vi "Lang Set Image Page.vi"(8 "error in (no error)":errorcluster, 10 "Image":T1, 11 "Configuration Window in":refnum<class "Configuration Window.lvclass">) -> (0 "error out":errorcluster, 3 "Configuration Window out":refnum<class "Configuration Window.lvclass">)   [LabVIEW 2018, in "Configuration Window.lvlib" / "Configuration Window.lvclass"]
uses:
  Configuration Window.lvclass
  Framework/Framework/Const Lang CfgWnd Image.ctl
  Framework/Framework/Const Lang Property.ctl
  Configuration Window.lvclass/Configuration Window.ctl
  Framework/Framework/Framework.lvclass
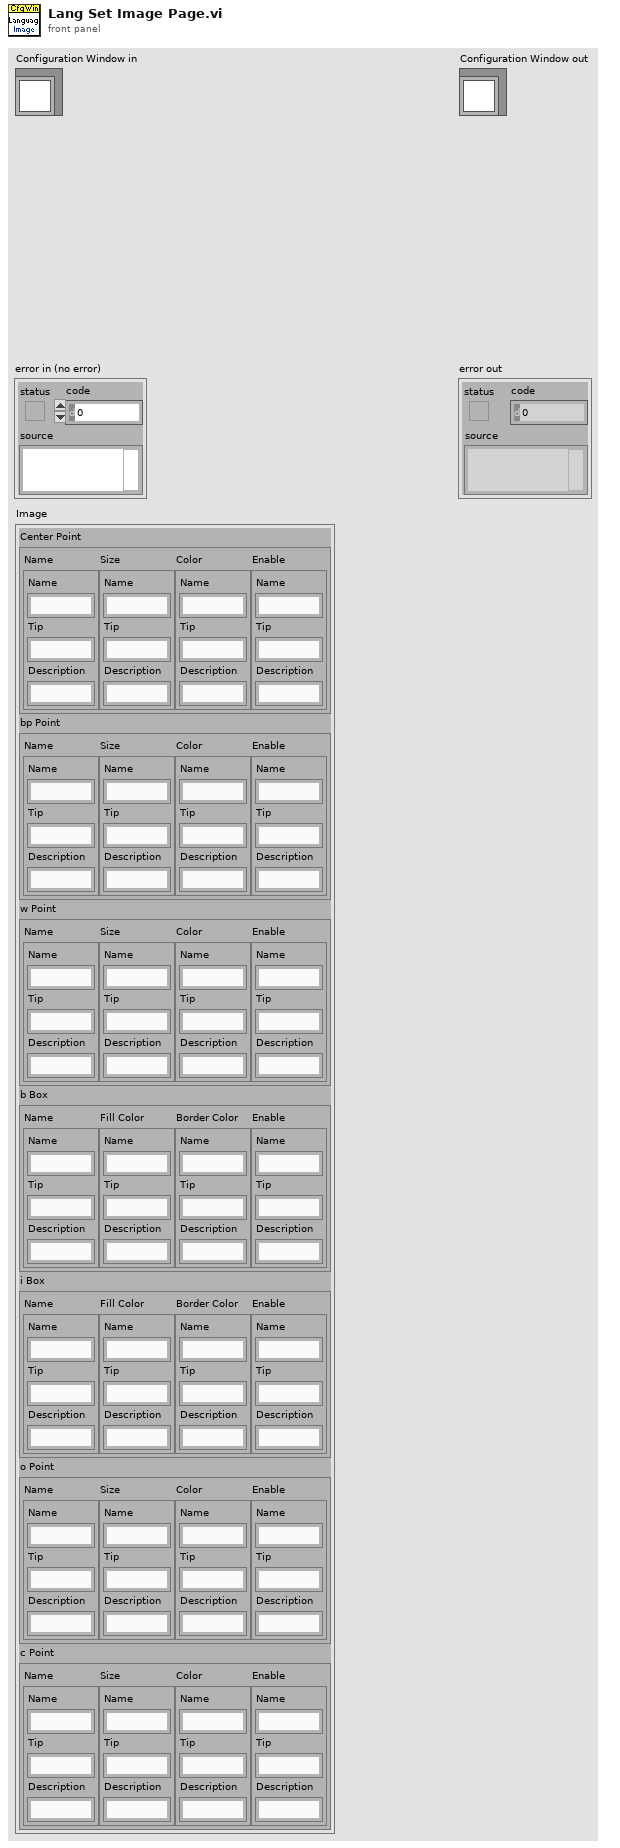
[diagram p1: front panel]
types:
  T1 = typedef "Framework.lvlib/Framework.lvclass/Const Lang CfgWnd Image.ctl" = cluster{"Center Point":cluster{"Name":T2, "Size":T2, "Color":T2, "Enable":T2}, "bp Point":cluster{"Name":T2, "Size":T2, "Color":T2, "Enable":T2}, "w Point":cluster{"Name":T2, "Size":T2, "Color":T2, "Enable":T2}, "b Box":cluster{"Name":T2, "Fill Color":T2, "Border Color":T2, "Enable":T2}, "i Box":cluster{"Name":T2, "Fill Color":T2, "Border Color":T2, "Enable":T2}, "o Point":cluster{"Name":T2, "Size":T2, "Color":T2, "Enable":T2}, "c Point":cluster{"Name":T2, "Size":T2, "Color":T2, "Enable":T2}}
  T2 = typedef "Framework.lvlib/Framework.lvclass/Const Lang Property.ctl" = cluster{"Name":string, "Tip":string, "Description":string}
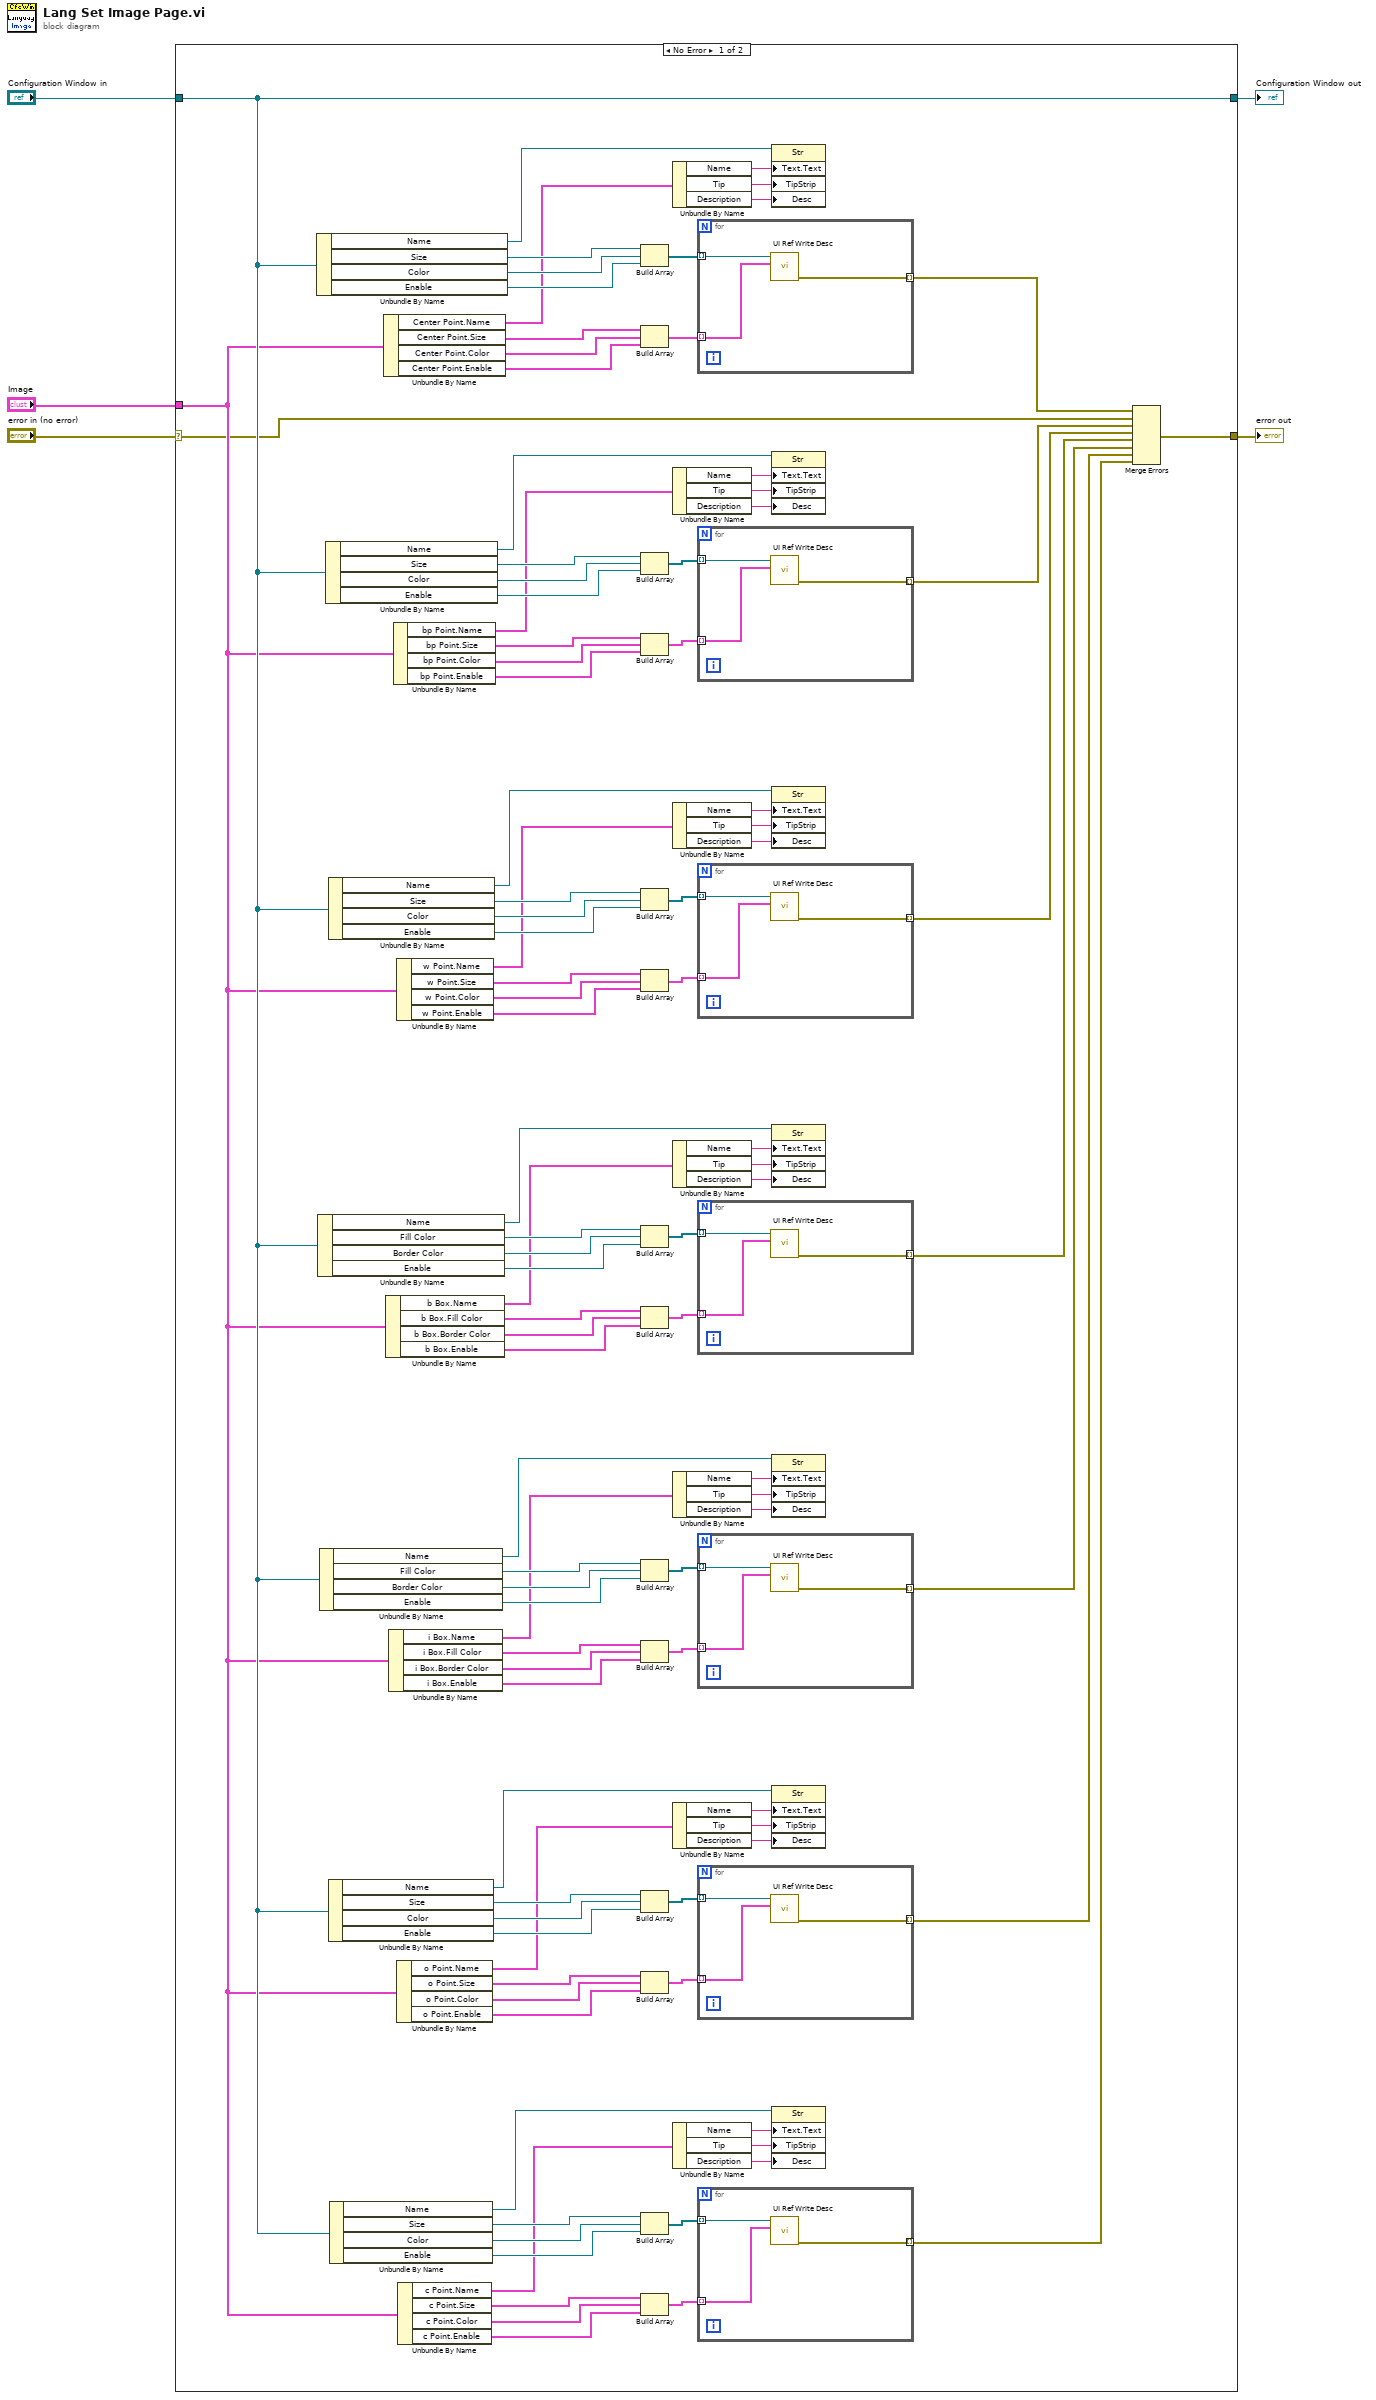
[diagram p0: block diagram]
diagram:
  n1 = case shown="No Error" "error in (no error)" {
    selector: "error in (no error)" -> [w41 w130]
    tunnel: [w106 w130] -> w4
    tunnel: [w55 w129] -> w2
    tunnel: "Configuration Window in" -> [w55 w129]
    tunnel: "Image" -> [w54 _]
    frame No Error {
      n2 = Unbundle By Name(w55) -> ("Name"=w40:refnum<vi>, "Size"=w105:refnum<vi>, "Color"=w104:refnum<vi>, "Enable"=w103:refnum<vi>)
      n3 = Unbundle By Name(w55) -> ("Name"=w22:refnum<vi>, "Fill Color"=w79:refnum<vi>, "Border Color"=w78:refnum<vi>, "Enable"=w77:refnum<vi>)
      n4 = Unbundle By Name(w55) -> ("Name"=w17:refnum<vi>, "Fill Color"=w71:refnum<vi>, "Border Color"=w70:refnum<vi>, "Enable"=w69:refnum<vi>)
      n5 = Unbundle By Name(w55) -> ("Name"=w33:refnum<vi>, "Size"=w95:refnum<vi>, "Color"=w94:refnum<vi>, "Enable"=w93:refnum<vi>)
      n6 = Unbundle By Name(w55) -> ("Name"=w27:refnum<vi>, "Size"=w87:refnum<vi>, "Color"=w86:refnum<vi>, "Enable"=w85:refnum<vi>)
      n7 = Unbundle By Name(w55) -> ("Name"=w12:refnum<vi>, "Size"=w63:refnum<vi>, "Color"=w62:refnum<vi>, "Enable"=w61:refnum<vi>)
      n8 = Unbundle By Name(w55) -> ("Name"=w7:refnum<vi>, "Size"=w53:refnum<vi>, "Color"=w52:refnum<vi>, "Enable"=w51:refnum<vi>)
      n9 = Unbundle By Name(w54) -> ("Center Point.Name"=w39:T2, "Center Point.Size"=w102:T2, "Center Point.Color"=w101:T2, "Center Point.Enable"=w100:T2)
      n10 = Unbundle By Name(w54) -> ("b Box.Name"=w21:T2, "b Box.Fill Color"=w76:T2, "b Box.Border Color"=w75:T2, "b Box.Enable"=w74:T2)
      n11 = Unbundle By Name(w54) -> ("i Box.Name"=w16:T2, "i Box.Fill Color"=w68:T2, "i Box.Border Color"=w67:T2, "i Box.Enable"=w66:T2)
      n12 = Unbundle By Name(w54) -> ("bp Point.Name"=w32:T2, "bp Point.Size"=w92:T2, "bp Point.Color"=w91:T2, "bp Point.Enable"=w90:T2)
      n13 = Unbundle By Name(w54) -> ("w Point.Name"=w26:T2, "w Point.Size"=w84:T2, "w Point.Color"=w83:T2, "w Point.Enable"=w82:T2)
      n14 = Unbundle By Name(w54) -> ("o Point.Name"=w11:T2, "o Point.Size"=w60:T2, "o Point.Color"=w59:T2, "o Point.Enable"=w58:T2)
      n15 = Unbundle By Name(w54) -> ("c Point.Name"=w6:T2, "c Point.Size"=w50:T2, "c Point.Color"=w49:T2, "c Point.Enable"=w48:T2)
      n16 = Build Array(w105, w104, w103) -> (w107:refnum<vi>[])
      n17 = Build Array(w102, w101, w100) -> (w99:T2[])
      n18 = Build Array(w95, w94, w93) -> (w96:refnum<vi>[])
      n19 = Build Array(w92, w91, w90) -> (w97:T2[])
      n20 = Build Array(w87, w86, w85) -> (w89:refnum<vi>[])
      n21 = Build Array(w84, w83, w82) -> (w88:T2[])
      n22 = Build Array(w79, w78, w77) -> (w80:refnum<vi>[])
      n23 = Build Array(w76, w75, w74) -> (w81:T2[])
      n24 = Build Array(w71, w70, w69) -> (w73:refnum<vi>[])
      n25 = Build Array(w68, w67, w66) -> (w72:T2[])
      n26 = Build Array(w63, w62, w61) -> (w64:refnum<vi>[])
      n27 = Build Array(w60, w59, w58) -> (w65:T2[])
      n28 = Build Array(w53, w52, w51) -> (w57:refnum<vi>[])
      n29 = Build Array(w50, w49, w48) -> (w56:T2[])
      n30 = Unbundle By Name(w39) -> ("Name"=w38:string, "Tip"=w37:string, "Description"=w36:string)
      n31 = Unbundle By Name(w32) -> ("Name"=w34:string, "Tip"=w35:string, "Description"=w31:string)
      n32 = Unbundle By Name(w26) -> ("Name"=w29:string, "Tip"=w28:string, "Description"=w30:string)
      n33 = Unbundle By Name(w21) -> ("Name"=w24:string, "Tip"=w25:string, "Description"=w23:string)
      n34 = Unbundle By Name(w16) -> ("Name"=w19:string, "Tip"=w18:string, "Description"=w20:string)
      n35 = Unbundle By Name(w11) -> ("Name"=w14:string, "Tip"=w15:string, "Description"=w13:string)
      n36 = Unbundle By Name(w6) -> ("Name"=w9:string, "Tip"=w8:string, "Description"=w10:string)
      n37 = for {
        tunnel: w107 -> [w128] mode=indexing
        tunnel: w99 -> [w127] mode=indexing
        tunnel: [w126] -> w98 mode=indexing
        n38 = call "UI Ref Write Desc.vi"("UI Property"=w127, "UI Ref"=w128) -> ("error out"=w126:errorcluster)  [unwired: 9 in]
      }
      n39 = for {
        tunnel: w96 -> [w125] mode=indexing
        tunnel: w97 -> [w124] mode=indexing
        tunnel: [w123] -> w47 mode=indexing
        n40 = call "UI Ref Write Desc.vi"("UI Property"=w124, "UI Ref"=w125) -> ("error out"=w123:errorcluster)  [unwired: 9 in]
      }
      n41 = for {
        tunnel: w89 -> [w121] mode=indexing
        tunnel: w88 -> [w120] mode=indexing
        tunnel: [w122] -> w46 mode=indexing
        n42 = call "UI Ref Write Desc.vi"("UI Property"=w120, "UI Ref"=w121) -> ("error out"=w122:errorcluster)  [unwired: 9 in]
      }
      n43 = for {
        tunnel: w80 -> [w118] mode=indexing
        tunnel: w81 -> [w117] mode=indexing
        tunnel: [w119] -> w45 mode=indexing
        n44 = call "UI Ref Write Desc.vi"("UI Property"=w117, "UI Ref"=w118) -> ("error out"=w119:errorcluster)  [unwired: 9 in]
      }
      n45 = for {
        tunnel: w73 -> [w115] mode=indexing
        tunnel: w72 -> [w114] mode=indexing
        tunnel: [w116] -> w44 mode=indexing
        n46 = call "UI Ref Write Desc.vi"("UI Property"=w114, "UI Ref"=w115) -> ("error out"=w116:errorcluster)  [unwired: 9 in]
      }
      n47 = for {
        tunnel: w64 -> [w112] mode=indexing
        tunnel: w65 -> [w111] mode=indexing
        tunnel: [w113] -> w43 mode=indexing
        n48 = call "UI Ref Write Desc.vi"("UI Property"=w111, "UI Ref"=w112) -> ("error out"=w113:errorcluster)  [unwired: 9 in]
      }
      n49 = for {
        tunnel: w57 -> [w109] mode=indexing
        tunnel: w56 -> [w108] mode=indexing
        tunnel: [w110] -> w42 mode=indexing
        n50 = call "UI Ref Write Desc.vi"("UI Property"=w108, "UI Ref"=w109) -> ("error out"=w110:errorcluster)  [unwired: 9 in]
      }
      n51 = property class="Str"(reference=w40, "Text.Text"=w38, "TipStrip"=w37, "Desc"=w36) -> ()  [unwired: 1 in, 2 out]
      n52 = property class="Str"(reference=w33, "Text.Text"=w34, "TipStrip"=w35, "Desc"=w31) -> ()  [unwired: 1 in, 2 out]
      n53 = property class="Str"(reference=w27, "Text.Text"=w29, "TipStrip"=w28, "Desc"=w30) -> ()  [unwired: 1 in, 2 out]
      n54 = property class="Str"(reference=w22, "Text.Text"=w24, "TipStrip"=w25, "Desc"=w23) -> ()  [unwired: 1 in, 2 out]
      n55 = property class="Str"(reference=w17, "Text.Text"=w19, "TipStrip"=w18, "Desc"=w20) -> ()  [unwired: 1 in, 2 out]
      n56 = property class="Str"(reference=w12, "Text.Text"=w14, "TipStrip"=w15, "Desc"=w13) -> ()  [unwired: 1 in, 2 out]
      n57 = property class="Str"(reference=w7, "Text.Text"=w9, "TipStrip"=w8, "Desc"=w10) -> ()  [unwired: 1 in, 2 out]
      n58 = Merge Errors(w98, w41, w47, w46, w45, w44, w43, w42) -> (w106:errorcluster)
    }
    frame Error {
    }
  }
  "error out" <- w4
  "Configuration Window out" <- w2
